vi "Register gRPC Methods.vi"(8 "error in (no error)":errorcluster, 11 "gRPC service in":refnum<class "Bus_Monitor_API.lvclass">) -> (0 "error out":errorcluster, 3 "gRPC service out":refnum<class "Bus_Monitor_API.lvclass">)   [LabVIEW 2026, in "bus_monitor_server.lvlib" / "Bus_Monitor_API.lvclass"]
uses:
  Bus_Monitor_API.lvclass
  Bus_Monitor_API.lvclass/Bus_Monitor_API.ctl
  typeDefs/Server Internal UEs.ctl
  typeDefs/Server gRPC UEs.ctl
  <vilib>/gRPC/LabVIEW gRPC Library/Shared/grpcId.ctl
  <vilib>/gRPC/LabVIEW gRPC Library/grpc-lvsupport-release.lvlib
  <vilib>/gRPC/LabVIEW gRPC Library/Server API/typeDefs/gRPCId Cluster.ctl
  typeDefs/Server Internal Message.ctl
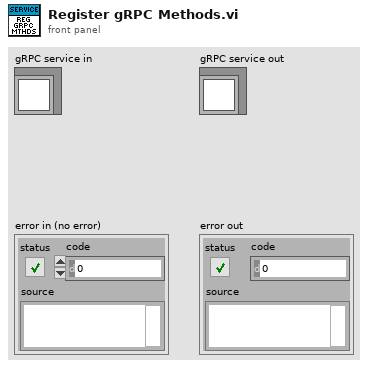
[diagram p1: front panel]
types:
  T1 = typedef "bus_monitor_server.lvlib/Bus_Monitor_API.lvclass/Server gRPC UEs.ctl" = cluster{"Bus_Monitor_API PassThru gRPC UE":refnum<user-event>, "Bus_Monitor_API GetStreamingFilter gRPC UE":refnum<user-event>, "Bus_Monitor_API SetStreamingFilter gRPC UE":refnum<user-event>, "Bus_Monitor_API ResetStreamingFilter gRPC UE":refnum<user-event>, "Bus_Monitor_API InitializeSettings gRPC UE":refnum<user-event>, "Bus_Monitor_API StopProcess gRPC UE":refnum<user-event>, "Bus_Monitor_API StreamBus gRPC UE":refnum<user-event>}
  T2 = typedef "bus_monitor_server.lvlib/Bus_Monitor_API.lvclass/Server Internal UEs.ctl" = cluster{"Bus_Monitor_API PassThru Internal UE":refnum<user-event>, "Bus_Monitor_API GetStreamingFilter Internal UE":refnum<user-event>, "Bus_Monitor_API SetStreamingFilter Internal UE":refnum<user-event>, "Bus_Monitor_API ResetStreamingFilter Internal UE":refnum<user-event>, "Bus_Monitor_API InitializeSettings Internal UE":refnum<user-event>, "Bus_Monitor_API StopProcess Internal UE":refnum<user-event>, "Bus_Monitor_API StreamBus Internal UE":refnum<user-event>}
  T3 = typedef "grpc-lvsupport-release.lvlib/grpcId.ctl" = u64
  T4 = typedef "bus_monitor_server.lvlib/Bus_Monitor_API.lvclass/Server Internal Message UE.ctl" = refnum<user-event>
  T5 = typedef "grpc-lvsupport-release.lvlib/gRPCId Cluster UE.ctl" = refnum<user-event>
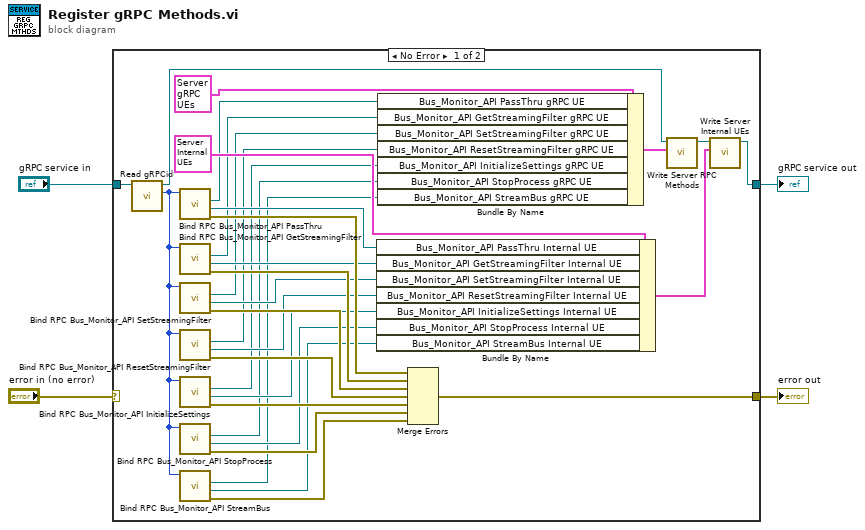
[diagram p0: block diagram]
diagram:
  n1 = case shown="No Error" "error in (no error)" {
    selector: "error in (no error)" -> [_ w36]
    tunnel: "gRPC service in" -> [w27 w37]
    tunnel: [w35 w36] -> w3
    tunnel: [w34 w37] -> w2
    frame No Error {
      n2 = call-dynamic "Read gRPCid.vi"("gRPC service in"=w27) -> ("gRPCid"=w26:T3, "gRPC service out"=w28:refnum<class "Bus_Monitor_API.lvclass">)  [unwired: 8 in, 1 out]
      n3 = call "Bind RPC Bus_Monitor_API PassThru.vi"("gRPCid server in"=w26) -> ("error out"=w25:errorcluster, "Bus_Monitor_API PassThru Internal UE"=w23:T4, "Bus_Monitor_API PassThru gRPC UE"=w24:T5)  [unwired: 7 in, 1 out]
      n4 = call "Bind RPC Bus_Monitor_API GetStreamingFilter.vi"("gRPCid server in"=w26) -> ("error out"=w22:errorcluster, "Bus_Monitor_API GetStreamingFilter Internal UE"=w20:T4, "Bus_Monitor_API GetStreamingFilter gRPC UE"=w21:T5)  [unwired: 7 in, 1 out]
      n5 = call "Bind RPC Bus_Monitor_API SetStreamingFilter.vi"("gRPCid server in"=w26) -> ("error out"=w19:errorcluster, "Bus_Monitor_API SetStreamingFilter Internal UE"=w17:T4, "Bus_Monitor_API SetStreamingFilter gRPC UE"=w18:T5)  [unwired: 7 in, 1 out]
      n6 = call "Bind RPC Bus_Monitor_API ResetStreamingFilter.vi"("gRPCid server in"=w26) -> ("error out"=w16:errorcluster, "Bus_Monitor_API ResetStreamingFilter Internal UE"=w14:T4, "Bus_Monitor_API ResetStreamingFilter gRPC UE"=w15:T5)  [unwired: 7 in, 1 out]
      n7 = call "Bind RPC Bus_Monitor_API InitializeSettings.vi"("gRPCid server in"=w26) -> ("error out"=w13:errorcluster, "Bus_Monitor_API InitializeSettings Internal UE"=w11:T4, "Bus_Monitor_API InitializeSettings gRPC UE"=w12:T5)  [unwired: 7 in, 1 out]
      n8 = call "Bind RPC Bus_Monitor_API StopProcess.vi"("gRPCid server in"=w26) -> ("error out"=w10:errorcluster, "Bus_Monitor_API StopProcess Internal UE"=w8:T4, "Bus_Monitor_API StopProcess gRPC UE"=w9:T5)  [unwired: 7 in, 1 out]
      n9 = call "Bind RPC Bus_Monitor_API StreamBus.vi"("gRPCid server in"=w26) -> ("error out"=w7:errorcluster, "Bus_Monitor_API StreamBus Internal UE"=w6:T4, "Bus_Monitor_API StreamBus gRPC UE"=w5:T5)  [unwired: 7 in, 1 out]
      n10 = Bundle By Name ("Bundle Internal UEs")(cluster=T2 {"Bus_Monitor_API PassThru Internal UE"=refnum, "Bus_Monitor_API GetStreamingFilter Internal UE"=refnum, "Bus_Monitor_API SetStreamingFilter Internal UE"=refnum, "Bus_Monitor_API ResetStreamingFilter Internal UE"=refnum, "Bus_Monitor_API InitializeSettings Internal UE"=refnum, "Bus_Monitor_API StopProcess Internal UE"=refnum, "Bus_Monitor_API StreamBus Internal UE"=refnum} ("Server Internal UEs"), "Bus_Monitor_API PassThru Internal UE"=w23, "Bus_Monitor_API GetStreamingFilter Internal UE"=w20, "Bus_Monitor_API SetStreamingFilter Internal UE"=w17, "Bus_Monitor_API ResetStreamingFilter Internal UE"=w14, "Bus_Monitor_API InitializeSettings Internal UE"=w11, "Bus_Monitor_API StopProcess Internal UE"=w8, "Bus_Monitor_API StreamBus Internal UE"=w6) -> (w33:T2)
      n11 = Bundle By Name ("Bundle gRPC UEs")(cluster=T1 {"Bus_Monitor_API PassThru gRPC UE"=refnum, "Bus_Monitor_API GetStreamingFilter gRPC UE"=refnum, "Bus_Monitor_API SetStreamingFilter gRPC UE"=refnum, "Bus_Monitor_API ResetStreamingFilter gRPC UE"=refnum, "Bus_Monitor_API InitializeSettings gRPC UE"=refnum, "Bus_Monitor_API StopProcess gRPC UE"=refnum, "Bus_Monitor_API StreamBus gRPC UE"=refnum} ("gRPC Server Method Events"), "Bus_Monitor_API PassThru gRPC UE"=w24, "Bus_Monitor_API GetStreamingFilter gRPC UE"=w21, "Bus_Monitor_API SetStreamingFilter gRPC UE"=w18, "Bus_Monitor_API ResetStreamingFilter gRPC UE"=w15, "Bus_Monitor_API InitializeSettings gRPC UE"=w12, "Bus_Monitor_API StopProcess gRPC UE"=w9, "Bus_Monitor_API StreamBus gRPC UE"=w5) -> (w30:T1)
      n12 = Merge Errors(w25, w22, w19, w16, w13, w10, w7) -> (w35:errorcluster)
      n13 = call "Write Server RPC Methods.vi"("Server RPC Methods"=w30, "gRPC service in"=w28) -> ("gRPC service out"=w31:refnum<class "Bus_Monitor_API.lvclass">)  [unwired: 8 in, 1 out]
      n14 = call "Write Server Internal UEs.vi"("Server Internal UEs"=w33, "gRPC service in"=w31) -> ("gRPC service out"=w34:refnum<class "Bus_Monitor_API.lvclass">)  [unwired: 8 in, 1 out]
    }
    frame Error {
    }
  }
  "error out" <- w3
  "gRPC service out" <- w2
